vi "configureHeartbeat.vi"(8 "error in (no error)":errorcluster, 10 "MonoHeartbeatConfig":T1={"Heartbeat Interval (s)"=1.0, "Heartbeat Timeout (s)"=5.0} {"Heartbeat Timeout (s)" min=0.5 max=60.0 step=0.1 format="%.1f"; "Heartbeat Interval (s)" min=0.1 max=10.0 step=0.1 format="%.1f"}, 11 "MonoClientCommunicator in":refnum<class "MonoClientCommunicator.lvclass">) -> (0 "error out":errorcluster, 3 "MonoClientCommunicator out":refnum<class "MonoClientCommunicator.lvclass">)   [LabVIEW 2016, in "MonoClientCommunicator.lvclass"]
uses:
  MonoClientCommunicator.lvclass
  ViewTest/MonoHeartbeat.ctl
  MonoClientCommunicator.lvclass/MonoClientCommunicator.ctl
  MonoHeartbeat/MonoHeartbeat.lvclass/MonoHeartbeat.ctl
  MonoHeartbeat/MonoHeartbeat.lvclass
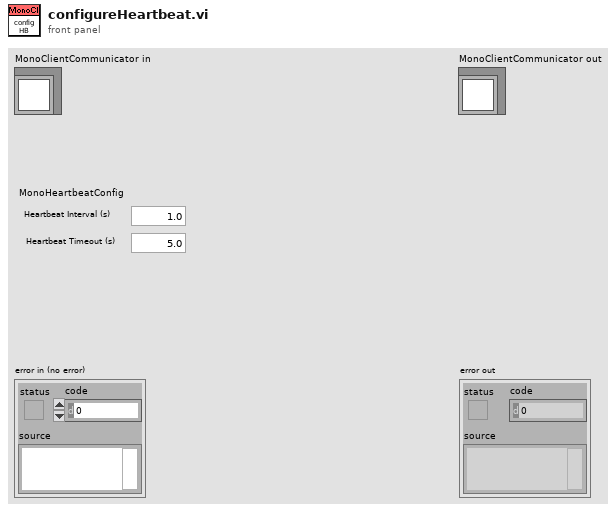
[diagram p1: front panel]
types:
  T1 = typedef "MonoHeartbeat.ctl" = cluster{"Heartbeat Interval (s)":dbl, "Heartbeat Timeout (s)":dbl}
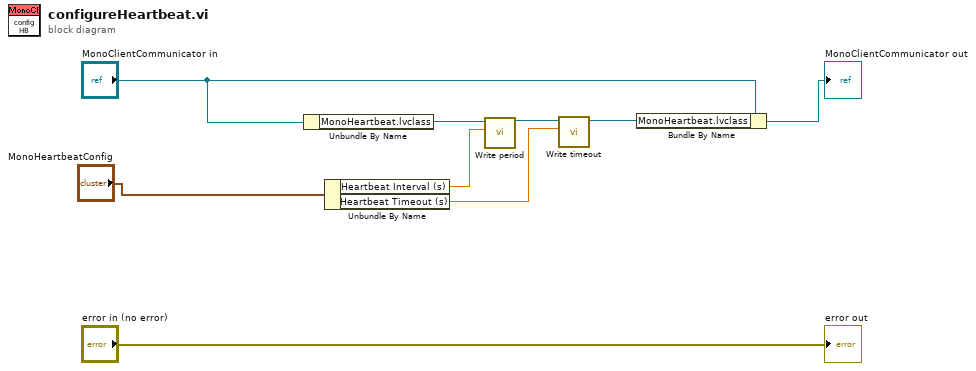
[diagram p0: block diagram]
diagram:
  n1 = Unbundle By Name("MonoClientCommunicator in") -> ("MonoHeartbeat.lvclass"=w5:refnum<class "MonoHeartbeat.lvclass">)
  n2 = Unbundle By Name("MonoHeartbeatConfig") -> ("Heartbeat Interval (s)"=w4:dbl, "Heartbeat Timeout (s)"=w3:dbl)
  n3 = call "Write period.vi"("period"=w4, "MonoHeartbeat in"=w5) -> ("MonoHeartbeat out"=w2:refnum<class "MonoHeartbeat.lvclass">)  [unwired: 8 in, 1 out]
  n4 = call "Write timeout.vi"("timeout"=w3, "MonoHeartbeat in"=w2) -> ("MonoHeartbeat out"=w1:refnum<class "MonoHeartbeat.lvclass">)  [unwired: 8 in, 1 out]
  n5 = Bundle By Name(cluster="MonoClientCommunicator in", "MonoHeartbeat.lvclass"=w1) -> (→"MonoClientCommunicator out":refnum<class "MonoClientCommunicator.lvclass">)
  "error out" <- "error in (no error)"
